vi "R-T测试.vi"   [LabVIEW 2019, in "test.lvlib"]
uses:
  test.lvlib
  <vilib>/Utility/file.llb/Read Delimited Spreadsheet (DBL).vi
  <vilib>/gmath/NI_Gmath.lvlib
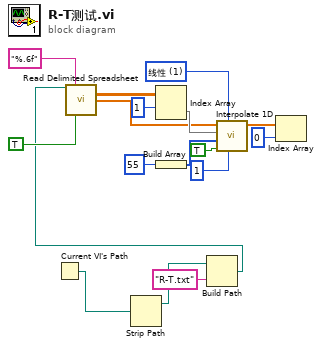
[diagram p0: block diagram]
diagram:
  w17 = 1 items=["最近", "线性", "样条", "cubic Hermite", "拉格朗日"] ("method")
  n1 = Current VI's Path() -> (path=w4:path)
  n2 = Strip Path(path=w4) -> (stripped path=w2:path)  [unwired: 1 out]
  n3 = Build Array(55) -> (w8:i32[])
  n4 = Build Path(base path=w2, name or relative path="R-T.txt" ("名称或相对路径")) -> (appended path=w1:path)
  n5 = call-poly <vilib>:"Read Delimited Spreadsheet.vi"("file path (dialog if empty)"=w1, "format (%.3f)"="%.6f", "transpose? (F)"=TRUE) -> ("all rows"=w14:dbl[][], "first row"=w11:dbl[])  [unwired: 7 in, 4 out]
  n6 = Index Array(array=w14, index (row)=1 ("索引 (行)")) -> (element=w12:dbl[])  [unwired: 1 in]
  n7 = call <vilib>:"Interpolate 1D.vi"("ntimes"=1, "method"=w17, "X is monotonic"=TRUE, "xi"=w8, "X"=w12, "Y"=w11) -> ("yi"=w7:dbl[])  [unwired: 3 in, 2 out]
  n8 = Index Array(array=w7, index=0 ("索引")) -> ()  [unwired: 1 out]
